vi "Actor Destroy.vi"(11 "Dev Actor in":refnum<class "Dev Actor.lvclass">) -> (0 "error out":errorcluster, 3 "Dev Actor out":refnum<class "Dev Actor.lvclass">)   [LabVIEW 2021, in "Dev Actor.lvlib" / "Dev Actor.lvclass"]
uses:
  Dev Actor.lvclass
  LVCAM/LVCAM/Msg Strategy/Msg Strategy.lvclass
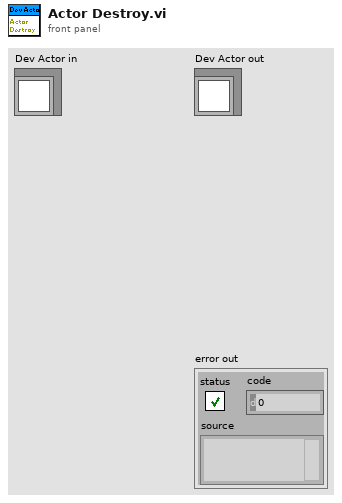
[diagram p1: front panel]
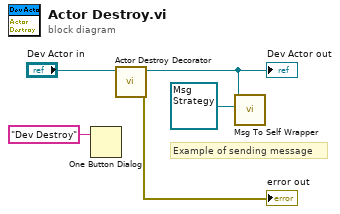
[diagram p0: block diagram]
diagram:
  # "Example of sending message"
  n1 = One Button Dialog(message="Dev Destroy") -> ()  [unwired: 1 in, 1 out]
  n2 = call "Actor Destroy Decorator.vi"("Dev Actor in"="Dev Actor in") -> ("error out"=→"error out":errorcluster, "Dev Actor out"=w2:refnum<class "Dev Actor.lvclass">)  [unwired: 9 in]
  "Dev Actor out" <- w2
  n3 = call "Msg To Self Wrapper.vi"("Msg"=refnum<class "Msg Strategy.lvclass"> refnum, "Dev Actor in"=w2) -> ()  [unwired: 9 in, 1 out]
